vi "_PC_Pub_MemoryofThisApp.vi"(1 "ThisApp Ref":refnum<vi>) -> (0 "number":dbl)   [LabVIEW 2018]
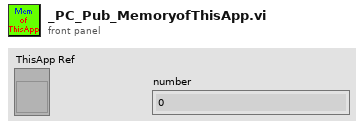
[diagram p1: front panel]
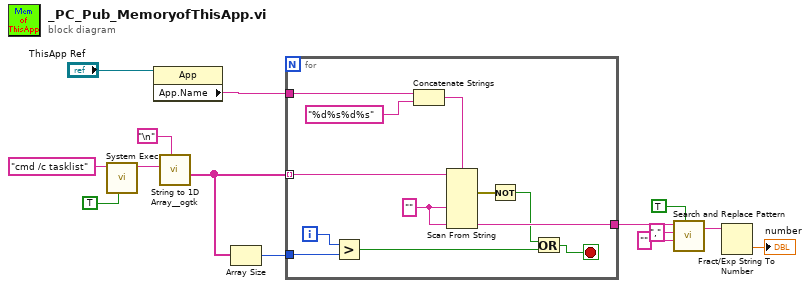
[diagram p0: block diagram]
diagram:
  n1 = call <vilib>:"System Exec.vi"("run minimized? (F)"=TRUE, "command line"="cmd /c tasklist") -> ("standard output"=w10:string)  [unwired: 6 in, 3 out]
  n2 = property class="App"(reference="ThisApp Ref") -> ("App.Name"=w11:string)  [unwired: 1 in, 2 out]
  n3 = call <userlib>:"String to 1D Array__ogtk.vi"("delimiter (Tab)"="\n", "string"=w10) -> ("Array of Strings"=w2:string[])  [unwired: 9 in]
  n4 = Array Size(array=w2) -> (size(s)=w1:i32)
  n5 = for {
    tunnel: w2 -> [w26] mode=indexing
    tunnel: w11 -> [w25]
    tunnel: [w21] -> w6
    tunnel: w1 -> [w19]
    i -> [w20]
    stop <- w15 stop-if-true
    w22 = ""
    n6 = Greater?(x=w20, y=w19) -> (0:w16:bool)
    n7 = Concatenate Strings(w25, "%d%s%d%s" ("string")) -> (w23:string)
    n8 = Scan From String(format string=w23, input string=w26, default 2=w22, default 4=w22) -> (error out=w18:errorcluster, output 4=w21:string)  [unwired: 7 in, 2 out]
    n9 = Not(x=w18) -> (.not. x?=w17:bool)
    n10 = Or(x=w17, y=w16) -> (x .or. y?=w15:bool)
  }
  n11 = call <vilib>:"Search and Replace Pattern.vi"("string"=w6, "regular expression (\"\")"="," ("regular expression (\"\")"), "replace string (\"\")"="" ("replace string (\"\")"), "replace all? (F)"=TRUE) -> ("result string"=w5:string)  [unwired: 1 in, 1 out]
  n12 = Fract/Exp String To Number(string=w5) -> (number=→"number":dbl)  [unwired: 3 in, 1 out]
